vi "FailureDescription.vi"(8 "error in (no error)":errorcluster, 10 "Actual":variant, 11 "Count in":refnum<class "Count.lvclass">) -> (0 "error out":errorcluster, 2 "Failure Description":string, 3 "Count out":refnum<class "Count.lvclass">)   [LabVIEW 2017, in "Transparent Assertions.lvlib" / "Constraints.lvlib" / "Count.lvclass"]
doc: "Return the second part of the scentence \"Failed asserting that ...\""
uses:
  Count.lvclass
  Count.lvclass/Count.ctl
  Constraints.lvlib
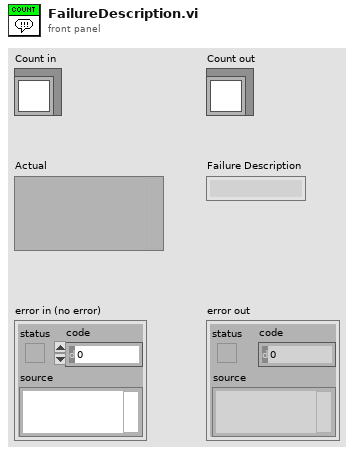
[diagram p1: front panel]
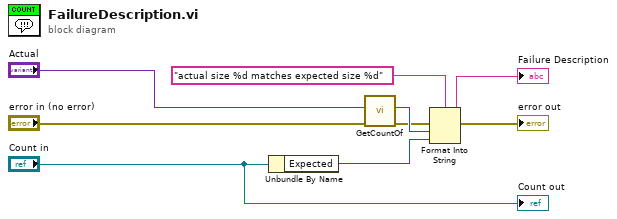
[diagram p0: block diagram]
diagram:
  n1 = Unbundle By Name("Count in") -> ("Expected"=w6:i32)
  n2 = call "GetCountOf.vi"("error in (no error)"="error in (no error)", "Countable"="Actual") -> ("error out"=w7:errorcluster, "Count"=w8:i32)  [unwired: 8 in]
  n3 = Format Into String(format string="actual size %d matches expected size %d", error in=w7, w8, w6) -> (resulting string=→"Failure Description":string, error out=→"error out":errorcluster)  [unwired: 1 in]
  "Count out" <- "Count in"
